vi "ordering state.vi"(4 "N_mech":u32=4, 5 "N":u32[](array[numeric])=[1, 1, 1, 1], 6 "Z3(State)":T2(array[ring])=[enum."stop ready", enum."stop ready", enum."stop ready", enum."stop ready"], 7 "Z1(CmdSource)":T1(array[ring])=[enum."auto", enum."auto", enum."auto", enum."auto"]) -> (0 "N_on":u32, 1 "N_ok":u32, 2 "OrderCoeff":u32[](array[numeric]), 3 "Order":u32[](array[numeric]))   [LabVIEW 2019, in "Userlib.lvlib"]
uses:
  Userlib.lvlib
panel:
  # "0 – выведен из работы по месту\n     1 – ручной местный\n     2 – ручной контроллера\n     3 – автомат контроллера\n     4 – дистационный"
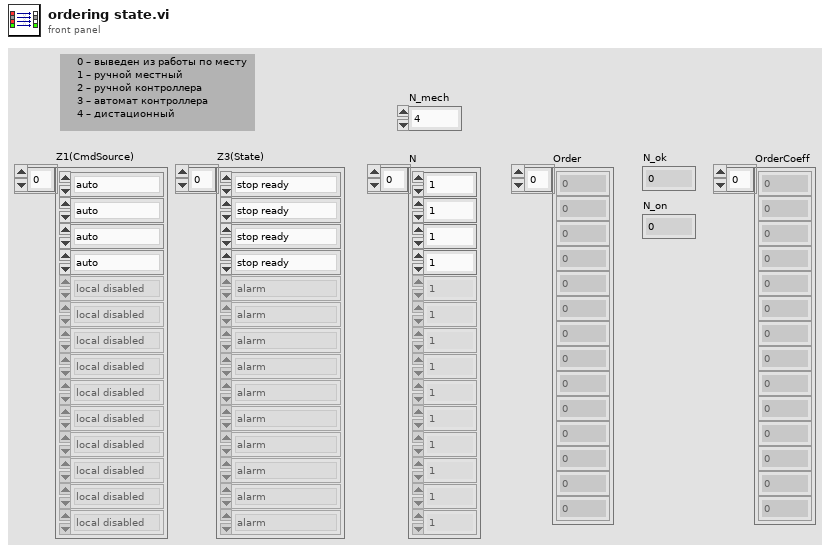
[diagram p1: front panel]
types:
  T1 = enum8{"local disabled", "local hand", "hand", "auto", "dist"}[]
  T2 = enum8{"alarm", "disabled", "not ready", "stop ready", "reserv", "switched off", "switched on", "check", "on min", "decrease speed", "on", "increase speed", "on max"}[]
  T3 = enum32{"local disabled", "local hand", "hand", "auto", "dist"}
  T4 = enum8{"local disabled", "local hand", "hand", "auto", "dist"}
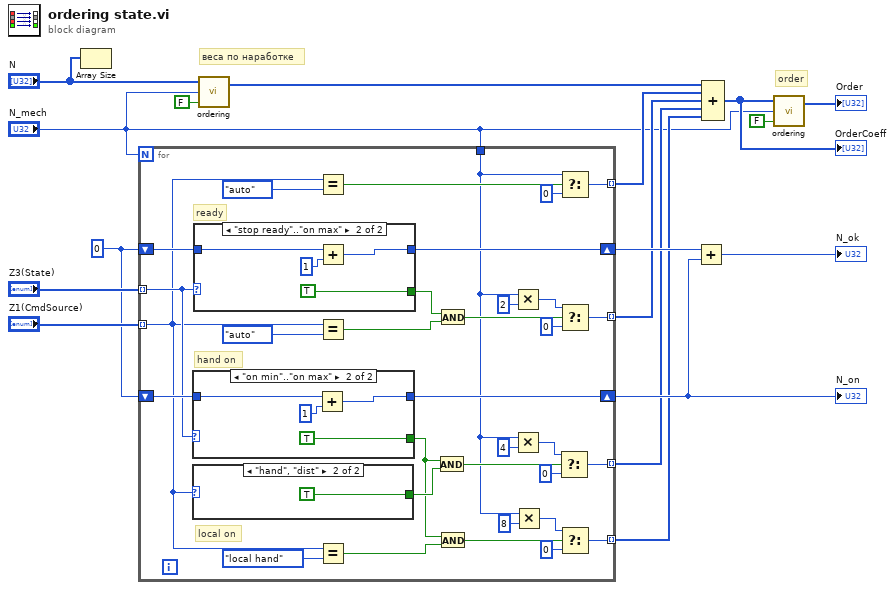
[diagram p0: block diagram]
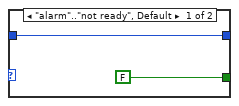
[diagram p2: hidden frame]
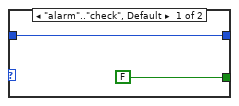
[diagram p3: hidden frame]
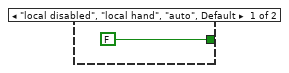
[diagram p4: hidden frame]
diagram:
  w12 = u32 0 ("y")
  # "order"
  # "веса по наработке"
  n1 = Array Size(array="N") -> ()  [unwired: 1 out]
  n2 = for {
    N: "N_mech" -> [_]
    tunnel: [w48] -> w5 mode=indexing
    tunnel: "Z3(State)" -> [w23] mode=indexing
    tunnel: [w46] -> w3 mode=indexing
    shift-right: [w29] -> w11
    shift-left: w12 -> [w28]
    tunnel: "N_mech" -> [w20]
    tunnel: "Z1(CmdSource)" -> [w18] mode=indexing
    shift-right: [w38] -> w9
    shift-left: w12 -> [w37]
    tunnel: [w36] -> w4 mode=indexing
    tunnel: [w19] -> w2 mode=indexing
    # "local on"
    # "hand on"
    # "ready"
    n3 = case shown="\"on min\"..\"on max\"" w23 {
      tunnel: [FALSE TRUE] -> w27
      tunnel: w37 -> [w57 w60]
      tunnel: [w57 w59] -> w38
      frame "alarm".."check", Default {
      }
      frame "on min".."on max" {
        n4 = Add(x=w60, y=u32 1) -> (x+y=w59:u32)
      }
    }
    n5 = case shown="\"hand\", \"dist\"" w18 {
      tunnel: [FALSE TRUE] -> w41
      frame "local disabled", "local hand", "auto", Default {
      }
      frame "hand", "dist" {
      }
    }
    n6 = case shown="\"stop ready\"..\"on max\"" w23 {
      tunnel: [FALSE TRUE] -> w30
      tunnel: w28 -> [w51 w54]
      tunnel: [w51 w53] -> w29
      frame "alarm".."not ready", Default {
      }
      frame "stop ready".."on max" {
        n7 = Add(x=w54, y=u32 1) -> (x+y=w53:u32)
      }
    }
    n8 = Equal?(x=w18, y=T3."auto" ("Z1(CmdSource)")) -> (x = y?=w21:bool)
    n9 = Equal?(x=w18, y=T3."auto" ("Z1(CmdSource)")) -> (x = y?=w32:bool)
    n10 = Equal?(x=w18, y=T4."local hand" ("Z1(CmdSource)")) -> (x = y?=w34:bool)
    n11 = And(x=w27, y=w41) -> (x .and. y?=w39:bool)
    n12 = And(x=w30, y=w32) -> (x .and. y?=w31:bool)
    n13 = And(x=w27, y=w34) -> (x .and. y?=w50:bool)
    n14 = Multiply(x=w20, y=u32 2) -> (x*y=w25:u32)
    n15 = Multiply(x=w20, y=u32 4) -> (x*y=w43:u32)
    n16 = Multiply(x=w20, y=u32 8) -> (x*y=w44:u32)
    n17 = Select(t=w43, s=w39, f=u32 0 ("y")) -> (s? t:f=w36:u32)
    n18 = Select(t=w20, s=w21, f=u32 0 ("y")) -> (s? t:f=w19:u32)
    n19 = Select(t=w25, s=w31, f=u32 0 ("y")) -> (s? t:f=w46:u32)
    n20 = Select(t=w44, s=w50, f=u32 0 ("y")) -> (s? t:f=w48:u32)
  }
  "N_on" <- w9
  n21 = call "ordering.vi"("Ascend"=FALSE, "N_mech"="N_mech", "N"="N") -> ("Order"=w7:u32[])  [unwired: 1 in]
  n22 = Add(x=w11, y=w9) -> (x+y=→"N_ok":u32)
  n23 = Compound Arithmetic op=ADD(w7, w2, w3, w4, w5) -> (w15:u32[])
  "OrderCoeff" <- w15
  n24 = call "ordering.vi"("Ascend"=FALSE, "N_mech"="N_mech", "N"=w15) -> ("Order"=→"Order":u32[])  [unwired: 1 in]
